vi "get_status.vi"(0 "reference (in)":i32, 5 "error in (no error)":errorcluster) -> (14 "reference (dup)":i32, 16 "motion_state":T1=enum."CONST", 17 "other_states":T1[](array[typedef]), 18 "status (raw result)":string, 19 "error out":errorcluster)   [LabVIEW 2012]
doc: "This VI retrieves the current status value(s) of the referenced device. There are two types of states the device can be in. One is a motion based state, where the device can be in only one of these states:\n\n(1) Idle (IDLE)\n(2) Running at constant speed (CONST)\n(3) Accelerating (ACCEL)\n(4) Decelerating (DECEL)\n\nThe other is non-motion based, where multiple states can exist at one time (in addition to the single motion state above)\n\nNOTE: if any of the following states exist in the \"other_states\" array output, then they are considered logically TRUE\n\n(1) Home input switch status (HOME_SWITCH)\n(2) Minus limit input switch status (-LIMIT_SWITCH)\n(3) Plus limit input switch status (+LIMIT_SWITCH)\n(4) Minus limit error (-LIMIT_ERR)\n(5) Plus limit error (+LIMIT_ERR)\n(6) Communication timeout counter alarm (COMM_ERR)\n\nProduced By:\n\nChristopher Lemieux\nKod Integrations, LLC\n4835 Marianne Drive\nMount Airy, MD 21771\nhttp://www.kodintegrations.com\nemail: clemieux@kodintegrations.com\nphone: (240) 687-1288"
uses:
  controls/status_states.ctl
  main_functions/commands.ctl
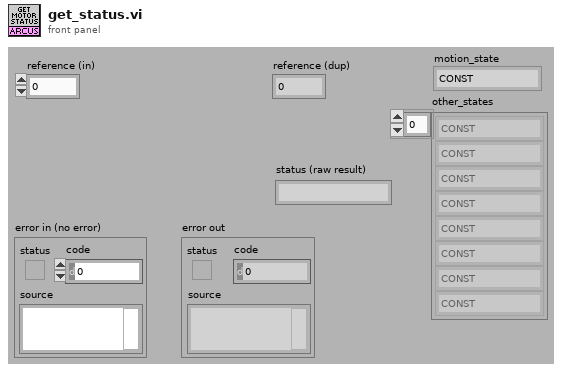
[diagram p1: front panel]
types:
  T1 = typedef "status_states.ctl" = enum16{"IDLE", "CONST", "ACCEL", "DECEL", "HOME_SWITCH", "-LIMIT_SWITCH", "+LIMIT_SWITCH", "-LIMIT_ERR", "+LIMIT_ERR", "COMM_ERR"}
  T2 = typedef "commands.ctl" = enum16{"clear error", "constant jog(-)", "constant jog(+)", "get acceleration", "get actual current", "get device id", "get digital input status", "get digial inputs status", "get dig output status", "get digital outputs status", "get firmware ver", "get high speed", "get idle current", "get low speed", "get micro step", "get motor status", "get move mode", "get polarity", "get position", "get product id", "get power status", "get run current", "get status", "home(-)", "home(+)", "move to position", "power down", "power up", "set acceleration", "set device id", "set digital output", "set digital outputs", "set high speed", "set idle current", "set low speed", "set move mode absolute", "set move mode increment", "set polarity", "set position", "set run current", "stop immediate", "stop slow", "store to memory"}
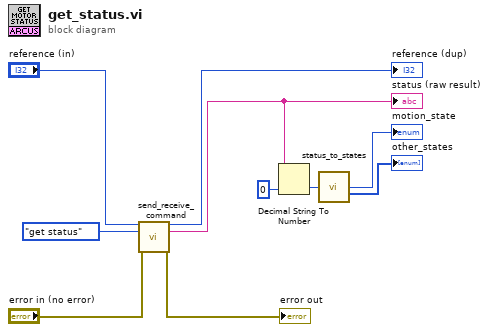
[diagram p0: block diagram]
diagram:
  n1 = call "send_receive_command.vi"("reference (in)"="reference (in)", "command"=commands."get status", "error in (no error)"="error in (no error)") -> ("reference (dup)"=→"reference (dup)":i32, "read_string"=w5:string, "error out"=→"error out":errorcluster)  [unwired: 8 in, 2 out]
  "status (raw result)" <- w5
  n2 = Decimal String To Number(string=w5, default (0L)=u32 0 ("default (0 I32)")) -> (number=w3:u32)  [unwired: 1 in, 1 out]
  n3 = call "status_to_states.vi"("actual value"=w3) -> ("motion_state"=→"motion_state":T1, "other_states"=→"other_states":T1[])  [unwired: 13 in]
